vi "emballage classe valve dans carton.vi"(0 "largeur index":i16, 1 "Offset début index":i16, 2 "Numéro du carton":i16, 3 "pc emballée/pc à emballer":string, 4 "Tab lot emballage":string[][](array[string])) -> (5 "chaîne tabulateur triée":string)   [LabVIEW 2020]
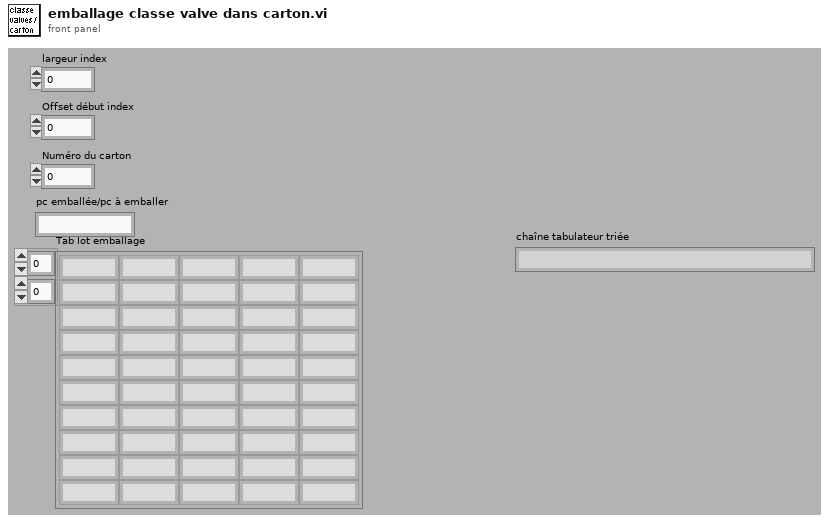
[diagram p1: front panel]
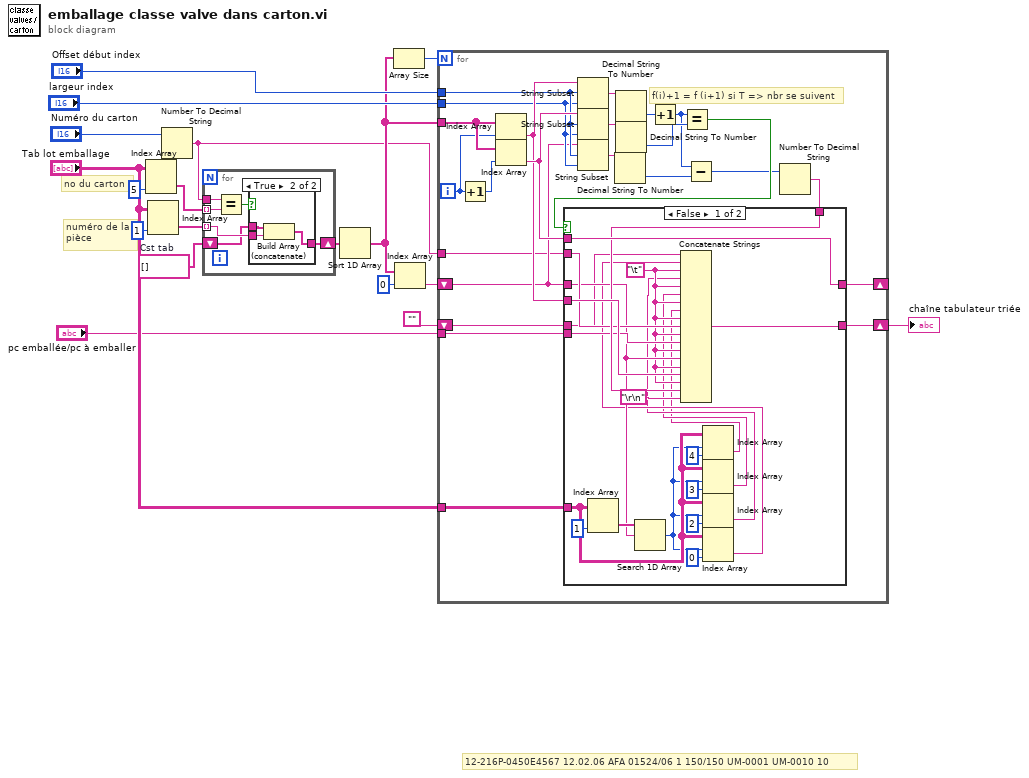
[diagram p0: block diagram]
diagram:
  w13 = string[] []  # Cst tab
  # "12-216P-0450E4567\t12.02.06\tAFA\t01524/06\t1\t150/150\tUM-0001\tUM-0010\t10"
  # "no du carton"
  # "numéro de la\npièce"
  n1 = Index Array(array="Tab lot emballage", index (col)=5) -> (element=w17:string[])  [unwired: 1 in]
  n2 = Index Array(array="Tab lot emballage", index (col)=1) -> (element=w15:string[])  [unwired: 1 in]
  n3 = Number To Decimal String(number="Numéro du carton") -> (decimal integer string=w4:string)  [unwired: 1 in]
  n4 = for {
    tunnel: w17 -> [w24] mode=indexing
    tunnel: w4 -> [w23]
    tunnel: w15 -> [w22] mode=indexing
    shift-right: [w21] -> w14
    shift-left: w13 -> [w20]
    n5 = Equal?(x=w23, y=w24) -> (x = y?=w19:bool)
    n6 = case shown="True" w19 {
      tunnel: w22 -> [_ w28]
      tunnel: [w25 w27] -> w21
      tunnel: w20 -> [w25 w26]
      frame False {
      }
      frame True {
        n7 = Build Array (concatenate)(w26, w28) -> (w27:string[])
      }
    }
  }
  n8 = Sort 1D Array(array=w14) -> (sorted array=w8:string[])
  n9 = Array Size(array=w8) -> (size(s)=w9:i32)
  n10 = Index Array(array=w8, index=0) -> (element=w7:string)
  n11 = for {
    N: w9 -> [_]
    tunnel: w8 -> [w49]
    tunnel: "Offset début index" -> [w39]
    tunnel: "largeur index" -> [w38]
    shift-right: [w45] -> _
    shift-left: w7 -> [w35]
    shift-right: [w42] -> w2
    shift-left: "" -> [w43]
    tunnel: "pc emballée/pc à emballer" -> [w31]
    tunnel: w4 -> [w30]
    tunnel: "Tab lot emballage" -> [w29]
    i -> [w48]
    # "f(i)+1 = f (i+1) si T => nbr se suivent"
    n12 = Increment(x=w48) -> (x+1=w47:i32)
    n13 = Index Array(array=w49, index=w48) -> (element=w41:string)
    n14 = Index Array(array=w49, index=w47) -> (element=w44:string)
    n15 = String Subset(string=w41, offset (0)=w39, length (rest)=w38) -> (substring=w52:string)
    n16 = String Subset(string=w44, offset (0)=w39, length (rest)=w38) -> (substring=w51:string)
    n17 = String Subset(string=w35, offset (0)=w39, length (rest)=w38) -> (substring=w37:string)
    n18 = Decimal String To Number(string=w37) -> (number=w36:i32)  [unwired: 2 in, 1 out]
    n19 = Decimal String To Number(string=w52) -> (number=w50:i32)  [unwired: 2 in, 1 out]
    n20 = Decimal String To Number(string=w51) -> (number=w40:i32)  [unwired: 2 in, 1 out]
    n21 = Increment(x=w50) -> (x+1=w33:i32)
    n22 = Equal?(x=w33, y=w40) -> (x = y?=w46:bool)
    n23 = Subtract(x=w33, y=w36) -> (x-y=w32:i32)
    n24 = Number To Decimal String(number=w32) -> (decimal integer string=w34:string)  [unwired: 1 in]
    n25 = case shown="False" w46 {
      tunnel: w35 -> [w65 w76]
      tunnel: [w74 w76] -> w45
      tunnel: w44 -> [w74 _]
      tunnel: w43 -> [w61 w75]
      tunnel: [w72 w75] -> w42
      tunnel: w41 -> [w73 _]
      tunnel: w34 -> [w70 _]
      tunnel: w31 -> [w69 _]
      tunnel: w30 -> [w68 _]
      tunnel: w29 -> [w55 _]
      frame False {
        w60 = "\t"
        n26 = Index Array(array=w55, index (col)=1) -> (element=w66:string[])  [unwired: 1 in]
        n27 = Search 1D Array(1D array=w66, element=w65) -> (index of element=w54:i32)  [unwired: 1 in]
        n28 = Index Array(array=w55, index (row)=w54, index (col)=4) -> (element=w53:string)
        n29 = Index Array(array=w55, index (row)=w54, index (col)=3) -> (element=w57:string)
        n30 = Index Array(array=w55, index (row)=w54, index (col)=2) -> (element=w58:string)
        n31 = Index Array(array=w55, index (row)=w54, index (col)=0) -> (element=w59:string)
        n32 = Concatenate Strings(w61, w59, w60, w58, w60, w57, w60, w53, w60, w68, w60, w69, w60, w65, w60, w73, w60, w70, "\r\n") -> (w72:string)
      }
      frame True {
      }
    }
  }
  "chaîne tabulateur triée" <- w2
